vi "lineFollowButton.vi"(7 "Right":bool, 8 "Middle":bool, 9 "Left":bool, 10 "Line Following Button":bool, 11 "Currently Line Following?":bool) -> (3 "Still Line Following?":bool)   [LabVIEW 2018]
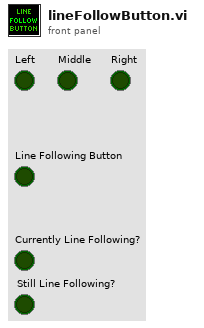
[diagram p1: front panel]
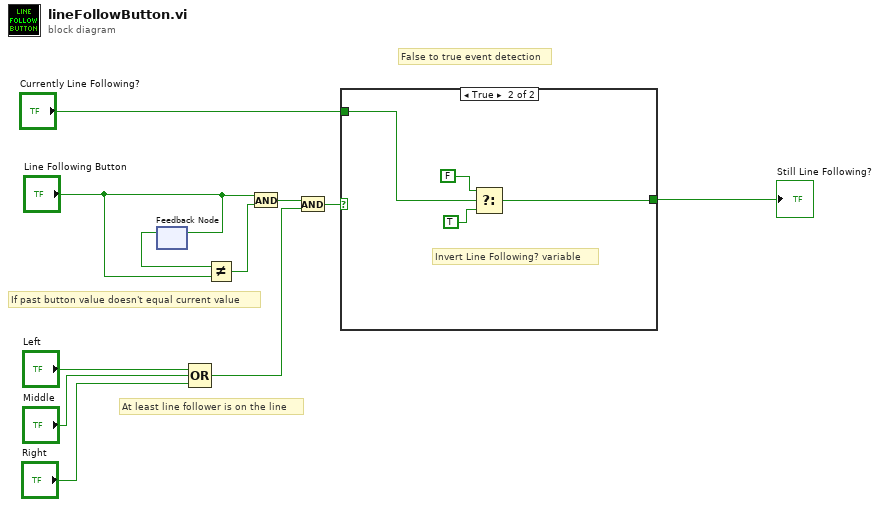
[diagram p0: block diagram]
diagram:
  # "At least line follower is on the line"
  # "If past button value doesn't equal current value"
  # "False to true event detection"
  n1 = feedback-in #1("Line Following Button") -> ()
  n2 = feedback #1() -> (w9:bool)  [unwired: 1 in]
  n3 = Compound Arithmetic op=OR("Left", "Middle", "Right") -> (w4:bool)
  n4 = Not Equal?(x=w9, y="Line Following Button") -> (x != y?=w11:bool)
  n5 = And(x="Line Following Button", y=w11) -> (x .and. y?=w6:bool)
  n6 = And(x=w6, y=w4) -> (x .and. y?=w5:bool)
  n7 = case shown="True" w5 {
    tunnel: [w12 w14] -> w7
    tunnel: "Currently Line Following?" -> [w12 w13]
    frame False {
      # "Do nothing"
    }
    frame True {
      # "Invert Line Following? variable"
      n8 = Select(t=FALSE, s=w13, f=TRUE) -> (s? t:f=w14:bool)
    }
  }
  "Still Line Following?" <- w7
